vi "Motion status.vi"(6 "Wait for updated value (F)":bool, 8 "error in":errorcluster, 9 "ms timeout (100)":i32=100) -> (0 "error out":errorcluster, 1 "timed out":bool, 2 "Motion status":T1={"Axis names"=["X", "Y", "Z", "Rx", "Ry", "Rz"], "Axis positions"=[], "Pose"=[], "Timestamp"=0, "Ready"=FALSE, "Stopped"=FALSE} {"Pose" format="%#.4f"; "Axis positions" format="%#.4f"}, 4 "timestamp":timestamp, 5 "quality":u64, 7 "status":u32)   [LabVIEW 2013]
uses:
  motion_status.ctl
panel:
  # "Read motion server status.   All the various arguments are for \"Datasocket Read\".  The default is to wait for up to 100 ms for an updated status.  To get the last published value, specify \"Wait for updated value\" false."
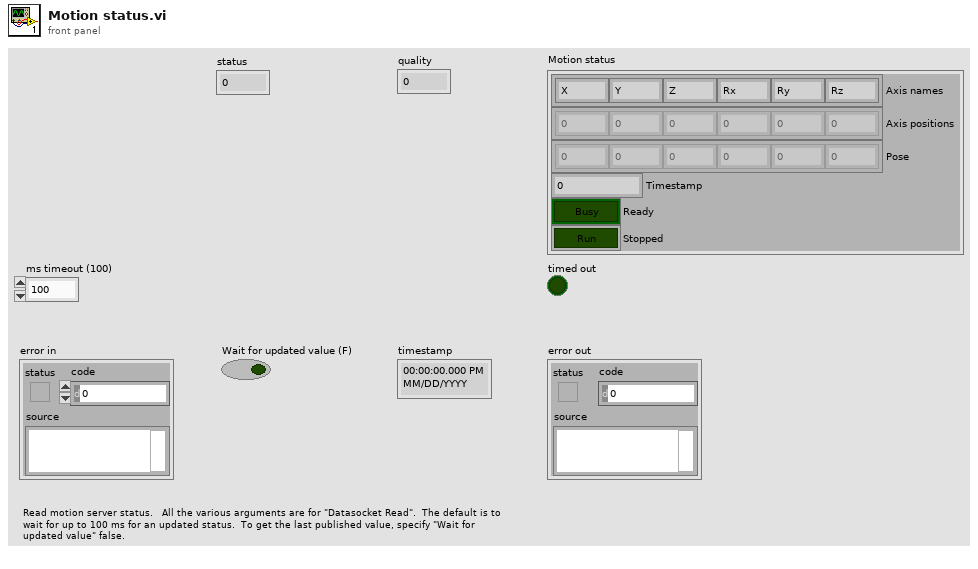
[diagram p1: front panel]
types:
  T1 = typedef "motion_status.ctl" = cluster{"Axis names":string[], "Axis positions":dbl[], "Pose":dbl[], "Timestamp":u32, "Ready":bool, "Stopped":bool}
  T2 = typedef "motion_variables.ctl" = cluster{"Motion command":refnum<k21>, "Motion status":refnum<k21>, "Emergency stop":refnum<k21>, "End transform":refnum<k21>, "Home position":refnum<k21>, "Axis offsets":refnum<k21>}
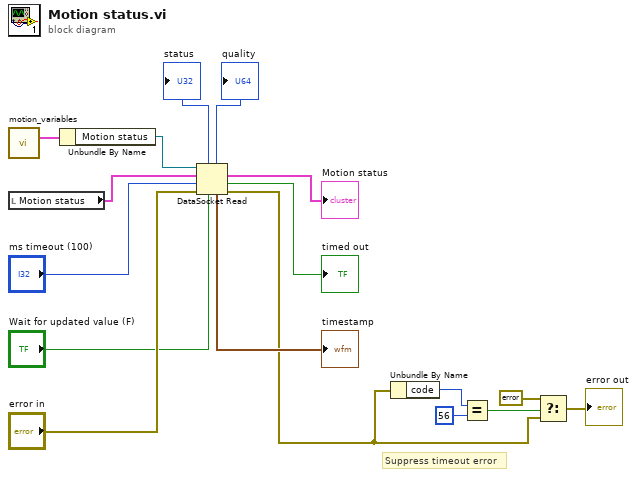
[diagram p0: block diagram]
diagram:
  # "Suppress timeout error"
  n1 = call "motion_variables.vi"() -> ("Motion variables"=w16:T2)  [unwired: 11 in]
  n2 = local read "Motion status"() -> (w7:T1)
  n3 = Unbundle By Name(w16) -> ("Motion status"=w17:refnum<k21>)
  n4 = DataSocket Read(6:"Wait for updated value (F)", 8:"error in", 9:"ms timeout (100)", 10:w7, 11:w17) -> (0:w3:errorcluster, 1:→"timed out":bool, 2:→"Motion status":T1, 4:→"timestamp":timestamp, 5:→"quality":u64, 7:→"status":u32)  [unwired: 1 out]
  n5 = Unbundle By Name(w3) -> ("code"=w6:i32)
  n6 = Equal?(x=w6, y=56) -> (x = y?=w4:bool)
  n7 = Select(t=errorcluster {"status"=FALSE, "code"=0, "source"=""}, s=w4, f=w3) -> (s? t:f=→"error out":errorcluster)
